vi "AlliGator Add Phasor Ratio to Plot.vi"(5 "New Plot Name":string, 7 "Plot ID (-1)":i32=-1, 8 "error in (no error)":errorcluster, 9 "Phasor Ratio":dbl, 10 "Abscissa":dbl, 11 "Phasor Ratio Graph refnum":refnum<vi>) -> (0 "error out":errorcluster, 1 "# Plots":i32, 2 "Actual Plot ID":i32, 3 "Phasor Ratio (dup)":dbl)   [LabVIEW 2021, in "AlliGator Phasor Ratio.lvlib"]
doc: "Adds single phasor ratio to a phasor ratio plot."
uses:
  AlliGator Phasor Ratio.lvlib
  Graphs/XY Graph/XY Graph Add-Ons.lvlib
panel:
  # "see the AlliGator License on the block diagram (Ctrl+E or Window:Show Block Diagram)"
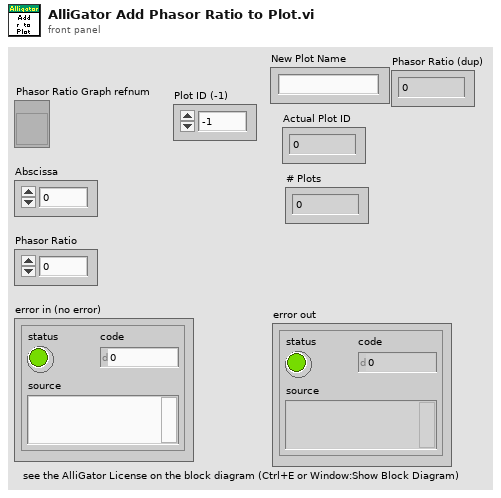
[diagram p1: front panel]
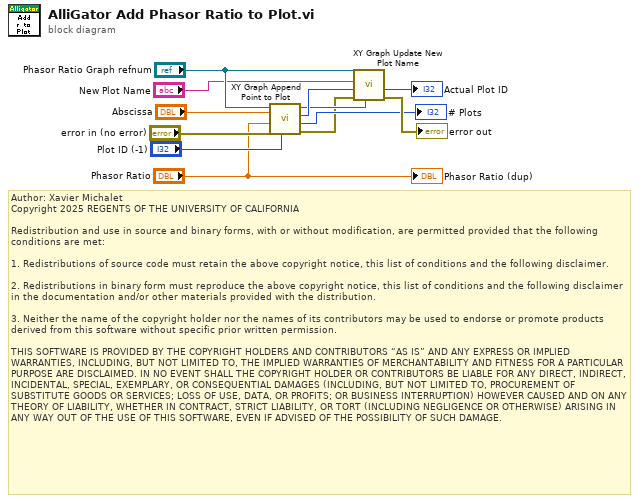
[diagram p0: block diagram]
diagram:
  # "Author: Xavier Michalet\nCopyright 2025 REGENTS OF THE UNIVERSITY OF CALIFORNIA\n\nRedistribution and use in source and binary forms, with or without modification, are permitted provided that the following conditions are met:\n\n1. Redistributions of source code must retain the above copyright notice, this list of conditions and the following disclaimer.\n\n2. Redistributions in binary form must reproduce the above copyright notice, this list of conditions and the following disclaimer in the documentation and/or other materials provided with the distribution.\n\n3. Neither the name of the copyright holder nor the names of its contributors may be used to endorse or promote products derived from this software without specific prior written permission.\n\nTHIS SOFTWARE IS PROVIDED BY THE COPYRIGHT HOLDERS AND CONTRIBUTORS “AS IS” AND ANY EXPRESS OR IMPLIED WARRANTIES, INCLUDING, BUT NOT LIMITED TO, THE IMPLIED WARRANTIES OF MERCHANTABILITY AND FITNESS FOR A PARTICULAR PURPOSE ARE DISCLAIMED. IN NO EVENT SHALL THE COPYRIGHT HOLDER OR CONTRIBUTORS BE LIABLE FOR ANY DIRECT, INDIRECT, INCIDENTAL, SPECIAL, EXEMPLARY, OR CONSEQUENTIAL DAMAGES (INCLUDING, BUT NOT LIMITED TO, PROCUREMENT OF SUBSTITUTE GOODS OR SERVICES; LOSS OF USE, DATA, OR PROFITS; OR BUSINESS INTERRUPTION) HOWEVER CAUSED AND ON ANY THEORY OF LIABILITY, WHETHER IN CONTRACT, STRICT LIABILITY, OR TORT (INCLUDING NEGLIGENCE OR OTHERWISE) ARISING IN ANY WAY OUT OF THE USE OF THIS SOFTWARE, EVEN IF ADVISED OF THE POSSIBILITY OF SUCH DAMAGE."
  n1 = call "XY Graph Append Point to Plot.vi"("Plot ID (-1: last)"="Plot ID (-1)", "error in (no error)"="error in (no error)", "y"="Phasor Ratio", "x"="Abscissa", "XYGraph in"="Phasor Ratio Graph refnum") -> ("error out"=w1:errorcluster, "# Plots"=→"# Plots":i32, "Actual Plot ID"=w7:i32, "Plot Created?"=w2:bool)  [unwired: 3 in]
  "Actual Plot ID" <- w7
  n2 = call "XY Graph Update New Plot Name.vi"("Plot Created?"=w2, "error in (no error)"=w1, "Actual Plot ID"=w7, "New Plot Name"="New Plot Name", "XYGraph in"="Phasor Ratio Graph refnum") -> ("error out"=→"error out":errorcluster)  [unwired: 6 in]
  "Phasor Ratio (dup)" <- "Phasor Ratio"
